vi "Subtract.vi"(7 "LabVIEW Web Service Request":refnum<class "Web Request.lvclass">) -> ()   [LabVIEW 2021]
uses:
  <vilib>/wsapi/Web Request.lvclass
panel:
  out "value":string
  out "c":dbl
  in  "B":dbl
  in  "A":dbl
  # "Use the Web Service Request input terminal to call the VIs on the Web Services palette. Do not remove it from the connector pane unless you don't need access to the palette."
  # "Each additional control wired to the connector pane will be available as an input in the URL. To include an indicator in terminal-mode output (the default setting), it must also be wired to the connector pane."
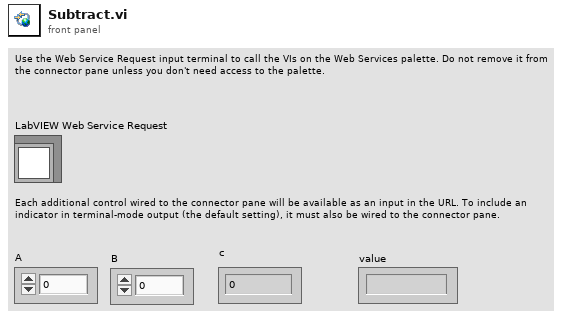
[diagram p1: front panel]
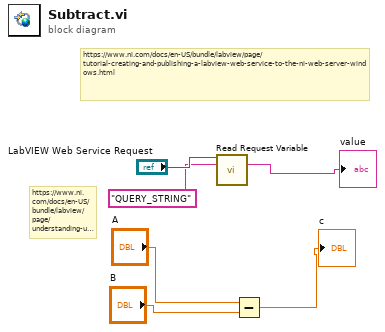
[diagram p0: block diagram]
diagram:
  # "https://www.ni.com/docs/en-US/bundle/labview/page/understanding-url-mappings-and-query-strings-in-web-services-real-time-windows.html"
  # "https://www.ni.com/docs/en-US/bundle/labview/page/tutorial-creating-and-publishing-a-labview-web-service-to-the-ni-web-server-windows.html"
  n1 = call <vilib>:"Read Request Variable.vi"("LabVIEW Web Service Request"="LabVIEW Web Service Request", "variable name"="QUERY_STRING") -> ("value"=→"value":string)  [unwired: 11 in, 2 out]
  n2 = Subtract(x="A", y="B") -> (x-y=→"c":dbl)
